vi "Get Data Variant.vi"(8 "error in":errorcluster, 11 "RDMA Rx Transfer Configuration in":refnum<class "RDMA Transfer Rx Configuration.lvclass">=refnum) -> (0 "error out":errorcluster, 1 "data version":T1, 2 "data":variant, 3 "RDMA Rx Transfer Configuration out":refnum<class "RDMA Transfer Rx Configuration.lvclass">)   [LabVIEW 2020, in "RDMA.lvlib" / "RDMA Transfer Rx Configuration.lvclass"]
uses:
  RDMA Transfer Rx Configuration.lvclass
  DSF Core.lvlibp/Typedefs/DSF Version Info.ctl
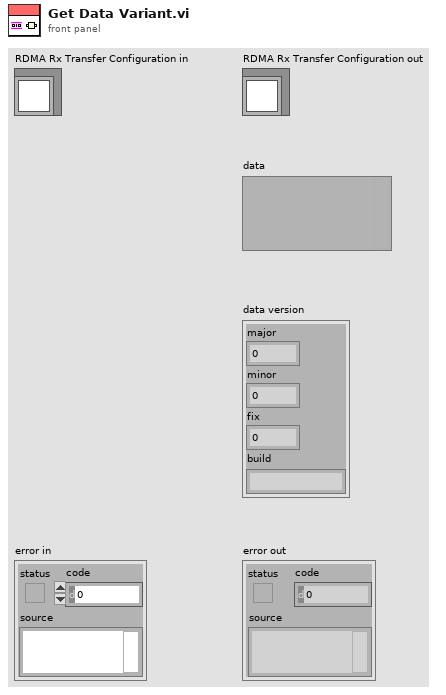
[diagram p1: front panel]
types:
  T1 = typedef "DSF Core.lvlibp/DSF Version Info.ctl" = cluster{"major":u32, "minor":u32, "fix":u32, "build":string}
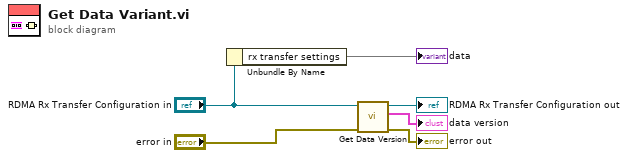
[diagram p0: block diagram]
diagram:
  n1 = Unbundle By Name("RDMA Rx Transfer Configuration in") -> ("rx transfer settings"=→"data")
  n2 = call-dynamic "Get Data Version.vi"("error in"="error in", "RDMA Rx Transfer Configuration in"="RDMA Rx Transfer Configuration in") -> ("error out"=→"error out":errorcluster, "data version"=→"data version":T1, "RDMA Rx Transfer Configuration out"=→"RDMA Rx Transfer Configuration out":refnum<class "RDMA Transfer Rx Configuration.lvclass">)  [unwired: 7 in]
